vi "Time Stamp.vi"(7 "key description":string, 8 "sections":string[](array[string]), 9 "time stamp":timestamp, 11 "info data":string) -> (0 "sections out":string[](array[string]), 3 "info data out":string)   [LabVIEW 2019, in "infolib.lvlib"]
doc: "Add a new date and time key to Info Data string. If section exists in Info Data string, inserts key into this section. If format is not set, ISO Date and Time format is used."
uses:
  infolib.lvlib
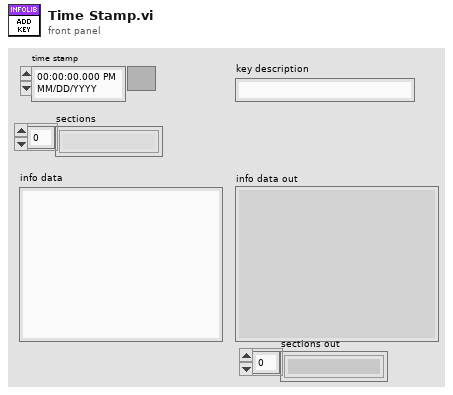
[diagram p1: front panel]
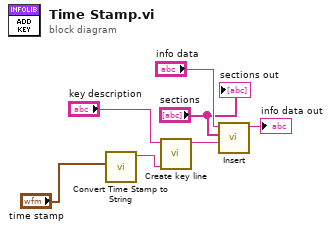
[diagram p0: block diagram]
diagram:
  n1 = call "Convert Time Stamp to String.vi"("time stamp"="time stamp") -> ("date/time string"=w3:string)  [unwired: 10 in]
  n2 = call "Create key line.vi"("formatted value"=w3, "key description"="key description") -> ("line"=w1:string)  [unwired: 9 in]
  n3 = call "Insert.vi"("insert"=w1, "sections"="sections", "info data"="info data") -> ("info data out"=→"info data out":string)  [unwired: 8 in]
  "sections out" <- "sections"
